vi "Filter Classes Descending from Test Casre.vi"(8 "error in (no error)":errorcluster, 11 "Project Items":refnum<vi>[](array[refnum])) -> (0 "error out":errorcluster, 3 "Project Items out":refnum<vi>[](array[refnum]))   [LabVIEW 2020, in "Coverage Analyzer.lvclass"]
uses:
  Coverage Analyzer.lvclass
  Coverage Analyzer.lvclass/Coverage Analyzer.ctl
  Test Case/LUnit Test Case.lvclass
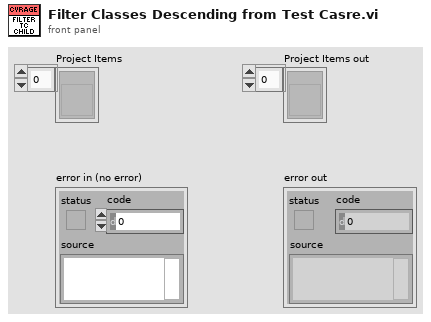
[diagram p1: front panel]
types:
  T1 = typedef "NI.Parent Library Information.ctl" = cluster{"qualified name":string, "localized name":string, "path":path, "parent library kind":T2}
  T2 = typedef "NI.Parent Library Kind.ctl" = enum32{"unknown", "class", "interface"}
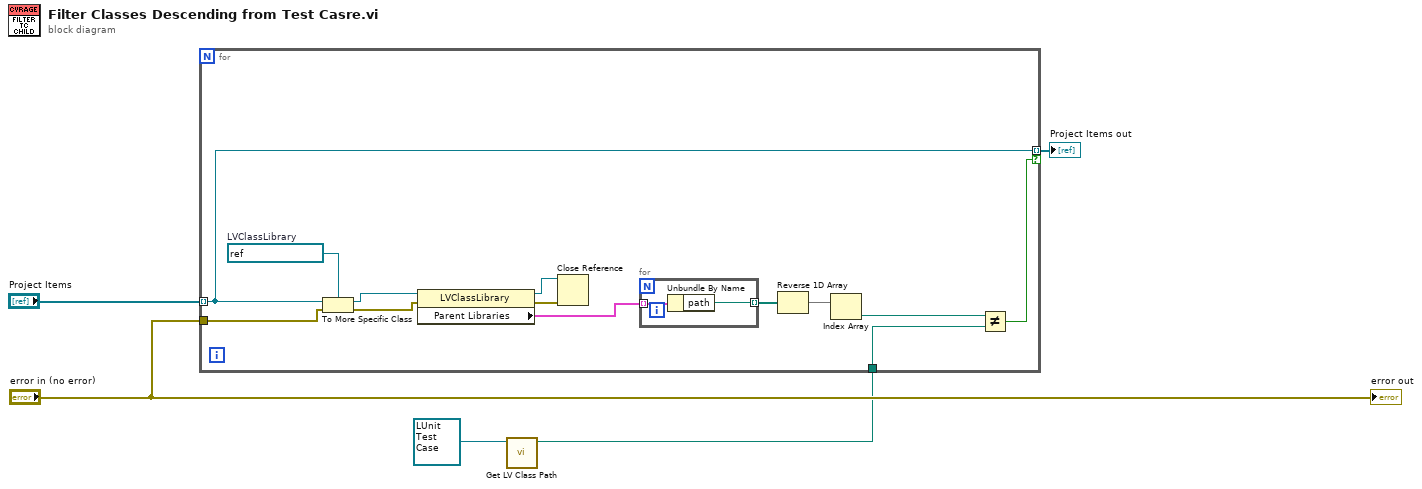
[diagram p0: block diagram]
diagram:
  n1 = call <vilib>:"Get LV Class Path.vi"("object"=refnum<class "LUnit Test Case.lvclass"> refnum ("LUnit Test Case.lvclass")) -> ("class path"=w2:path)  [unwired: 9 in, 1 out]
  n2 = for {
    tunnel: "Project Items" -> [w7] mode=indexing
    tunnel: "error in (no error)" -> [w18]
    tunnel: w2 -> [w9]
    tunnel: [w7] -> w1 mode=indexing if=w6
    w17 = refnum<vi> refnum  # LVClassLibrary
    n3 = To More Specific Class(target class=w17, reference=w7, error in=w18) -> (specific class reference=w15:refnum<vi>, error out=w14:errorcluster)
    n4 = property class="LVClassLibrary"(reference=w15, error in=w14) -> (reference out=w8:refnum<vi>, error out=w16:errorcluster, "Parent Libraries"=w10:T1[])
    n5 = Close Reference(reference=w8, error in (no error)=w16) -> ()  [unwired: 1 out]
    n6 = for {
      tunnel: w10 -> [w20] mode=indexing
      tunnel: [w19] -> w11 mode=indexing
      n7 = Unbundle By Name(w20) -> ("path"=w19:path)
    }
    n8 = Reverse 1D Array(array=w11) -> (reversed array=w13:path[])
    n9 = Index Array(array=w13) -> (element=w12:path)  [unwired: 1 in]
    n10 = Not Equal?(x=w12, y=w9) -> (x != y?=w6:bool)
  }
  "Project Items out" <- w1
  "error out" <- "error in (no error)"
